vi "Final_UI.vi"() -> ()   [LabVIEW 2020]
panel:
  in  "VISA resource name":refnum<visa-resource-name>
  in  "Table Control":string[][](table)
  out "Humidity":dbl(graph)
  out "Temperature":i32(graph)
  out "Humidity":dbl(knob) scale=0.0..100.0
  out "Thermometer":dbl(slide) scale=0.0..50.0
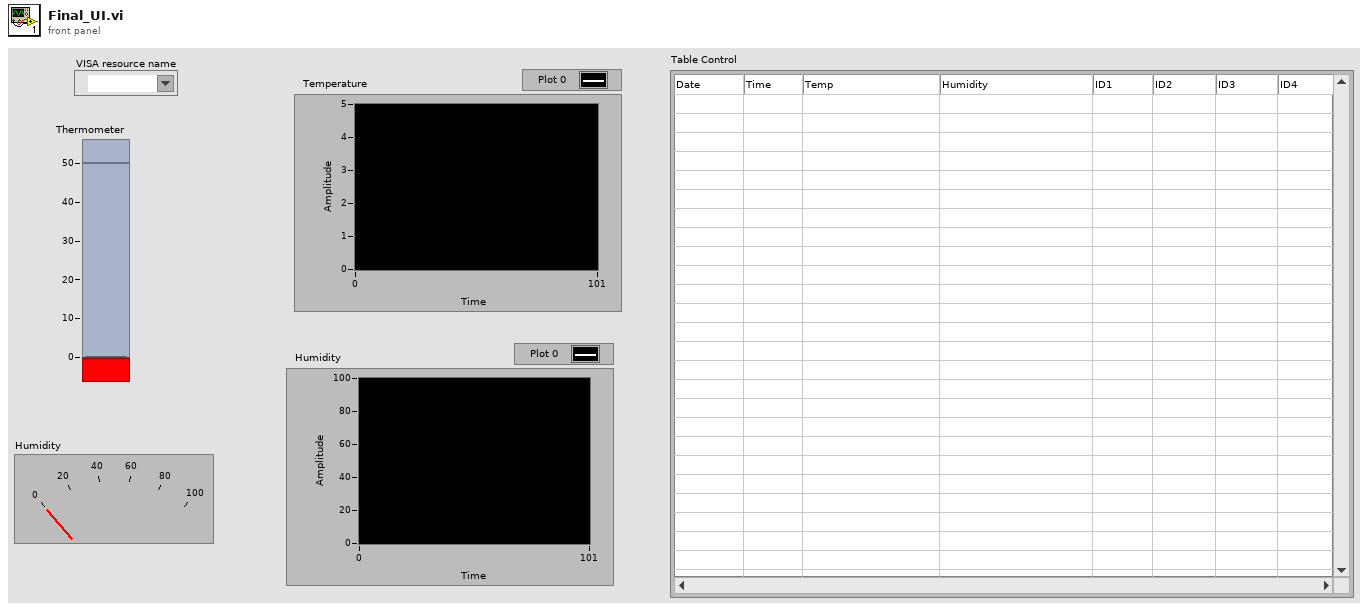
[diagram p1: front panel]
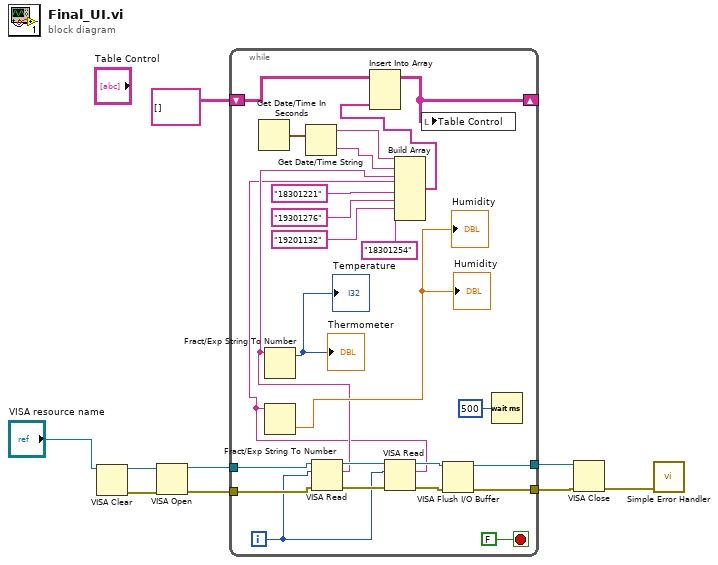
[diagram p0: block diagram]
diagram:
  n1 = VISA Clear(VISA resource name="VISA resource name") -> (VISA resource name out=w8:refnum<visa-resource-name>, error out=w9:errorcluster)  [unwired: 1 in]
  n2 = VISA Open(error in (no error)=w9, VISA resource name=w8) -> (VISA resource name=w6:refnum<visa-resource-name>, error out=w4:errorcluster)  [unwired: 3 in]
  n3 = while {
    tunnel: w6 -> [w34]
    tunnel: [w31] -> w5
    tunnel: w4 -> [w30]
    tunnel: [w27] -> w3
    shift-right: [w23] -> _
    shift-left: string[][] [] -> [w24]
    i -> [w26]
    stop <- FALSE stop-if-true
    n4 = Get Date/Time In Seconds() -> (seconds since 1Jan1904=w19:timestamp)
    n5 = Get Date/Time String(seconds (now)=w19) -> (date string=w21:string, time string=w20:string)  [unwired: 2 in]
    n6 = VISA Read(VISA resource name=w34, byte count=w26, error in (no error)=w30) -> (VISA resource name out=w33:refnum<visa-resource-name>, read buffer=w15:string, error out=w29:errorcluster)  [unwired: 1 out]
    n7 = Fract/Exp String To Number(string=w15) -> (offset past number=→"Thermometer" →"Temperature":i32)  [unwired: 3 in, 1 out]
    n8 = VISA Read(VISA resource name=w33, byte count=w26, error in (no error)=w29) -> (VISA resource name out=w32:refnum<visa-resource-name>, read buffer=w14:string, error out=w28:errorcluster)  [unwired: 1 out]
    n9 = Fract/Exp String To Number(string=w14) -> (number=→"Humidity" →"Humidity":dbl)  [unwired: 3 in, 1 out]
    n10 = Build Array(w21, w20, w15, w14, "18301221" ("element"), "19301276" ("element"), "19201132" ("element"), "18301254" ("element")) -> (w18:string[])
    n11 = Insert Into Array(array=w24, new element=w18) -> (w23:string[][])  [unwired: 2 in]
    n12 = local write "Table Control"(w23) -> ()
    n13 = VISA Flush I/O Buffer(VISA resource name=w32, error in (no error)=w28) -> (VISA resource name out=w31:refnum<visa-resource-name>, error out=w27:errorcluster)  [unwired: 1 in]
    n14 = Wait (ms)(milliseconds to wait=u32 500) -> ()  [unwired: 1 out]
  }
  n15 = VISA Close(VISA resource name=w5, error in (no error)=w3) -> (error out=w7:errorcluster)
  n16 = call <vilib>:"Simple Error Handler.vi"("error in (no error)"=w7) -> ()  [unwired: 4 in, 5 out]
